vi "Debug_main.vi"() -> ()   [LabVIEW 2025]
uses:
  <vilib>/jgoebel/LabVIEW MCP Server SDK/MCP Server.lvlibp
panel:
  out "Numeric":i32
  in  "stop":bool
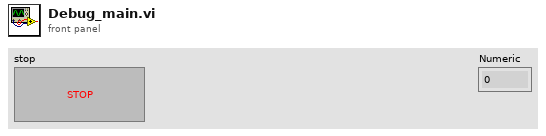
[diagram p1: front panel]
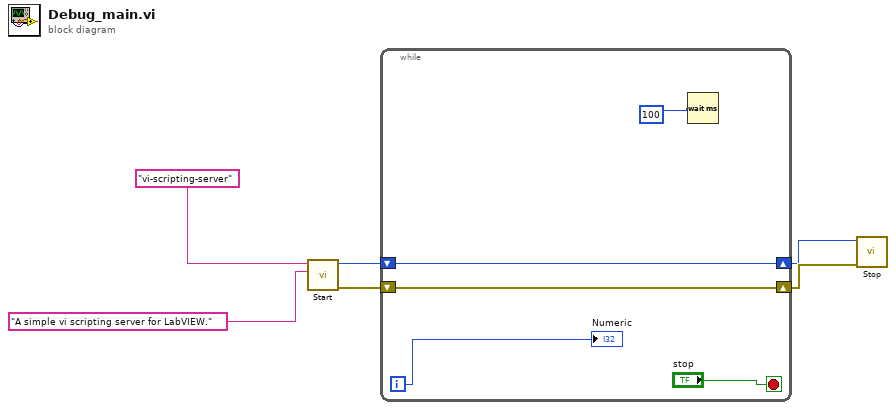
[diagram p0: block diagram]
diagram:
  n1 = call <vilib>:"Start.vi"("Description"="A simple vi scripting server for LabVIEW.", "Name"="vi-scripting-server") -> ("error out"=w6:errorcluster, "id out"=w4:i32)  [unwired: 7 in, 1 out]
  n2 = while {
    shift-right: [w11] -> w5
    shift-left: w6 -> [w11]
    shift-right: [w10] -> w3
    shift-left: w4 -> [w10]
    i -> [w8]
    stop <- "stop" stop-if-true
    n3 = Wait (ms)(milliseconds to wait=u32 100) -> ()  [unwired: 1 out]
    "Numeric" <- w8
  }
  n4 = call <vilib>:"Stop.vi"("error in (no error)"=w5, "id"=w3) -> ()  [unwired: 9 in, 1 out]
